vi "Start Module.vi"(6 "Show Main VI Diagram on Init (F)":bool, 8 "error in (no error)":errorcluster, 9 "DB-Engine":refnum<class "DB-Interface.lvclass">, 10 "Config Section":string, 11 "Run as Singleton? (F)":bool) -> (0 "error out":errorcluster, 1 "Wait for Event Sync?":bool, 2 "DB_CONNECTOR Broadcast Events":T1, 3 "Module ID":i32)   [LabVIEW 2022 SP3, in "hse-db.lvlib" / "DB_CONNECTOR.lvlib"]
doc: "Launches the Module Main.vi.\n____\nHAMPEL SOFTWARE ENGINEERING v1.4.0 (2023-12-19 09:52)"
uses:
  DB_CONNECTOR.lvlib
  Broadcast Events--cluster.ctl
  Did Init Argument--cluster.ctl
  Status Updated Argument--cluster.ctl
  Error Reported Argument--cluster.ctl
  Stop Argument--cluster.ctl
  Get Module Execution Status Argument--cluster.ctl
  Fast Query Reply Argument--cluster.ctl
  Configured and Connected Argument--cluster.ctl
  DB-Interface/DB-Interface.lvclass
  Module Running State--enum.ctl
  <vilib>/Delacor/Delacor QMH/Libraries/Cloneable Module Admin_class/Delacor_lib_QMH_Cloneable Module Admin.lvclass
  C:/Program Files/National Instruments/LabVIEW 2022/vi.lib/Delacor/Delacor QMH/Libraries/Module Admin_class/Delacor_lib_QMH_Module Admin.lvclass
  VI Reference Management/Main VI Type--strict_vi_ref.ctl
  <vilib>/Delacor/Delacor QMH/Libraries/Cloneable Module Admin_class/Delacor_lib_QMH_Cloneable Module Admin.lvclass/Delacor_lib_QMH_Cloneable Module Admin.ctl
  <vilib>/Delacor/Delacor QMH/Libraries/Module Admin_class/Delacor_lib_QMH_Module Admin.lvclass/Delacor_lib_QMH_Module Admin.ctl
  <vilib>/Delacor/Delacor QMH/Libraries/Cloneable Module Admin_class/Delacor_lib_QMH_Set Module ID.vi
  <vilib>/Delacor/Delacor QMH/Libraries/Module Admin_class/Delacor_lib_QMH_Set External Launch.vi
  Main.vi
  <vilib>/Utility/error.llb/Error Cluster From Error Code.vi
  <vilib>/ErrorRing/Error Ring.xnode
  Clone Registration/Clone Registration.lvlib
  VI Reference Management/VI Reference Management.lvlib
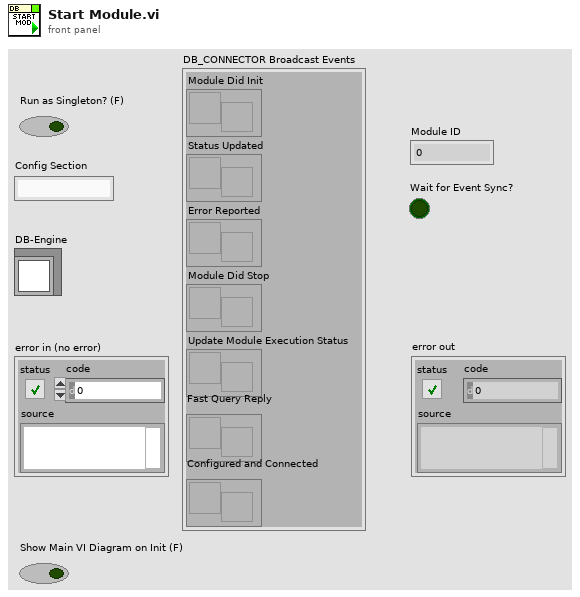
[diagram p1: front panel]
types:
  T1 = typedef "hse-db.lvlib/DB_CONNECTOR.lvlib/Broadcast Events--cluster.ctl" = cluster{"Module Did Init":refnum<user-event>, "Status Updated":refnum<user-event>, "Error Reported":refnum<user-event>, "Module Did Stop":refnum<user-event>, "Update Module Execution Status":refnum<user-event>, "Fast Query Reply":refnum<user-event>, "Configured and Connected":refnum<user-event>}
  T2 = typedef "hse-db.lvlib/DB_CONNECTOR.lvlib/Module Running State--enum.ctl" = enum16{"Not Running", "Running as Cloneable", "Running as Singleton"}
  T3 = enum32{"Bad", "Idle", "Run top level", "Running"}
  T4 = typedef "hse-db.lvlib/DB_CONNECTOR.lvlib/VI Reference Management.lvlib/Main VI Type--strict_vi_ref.ctl" = refnum<vi>
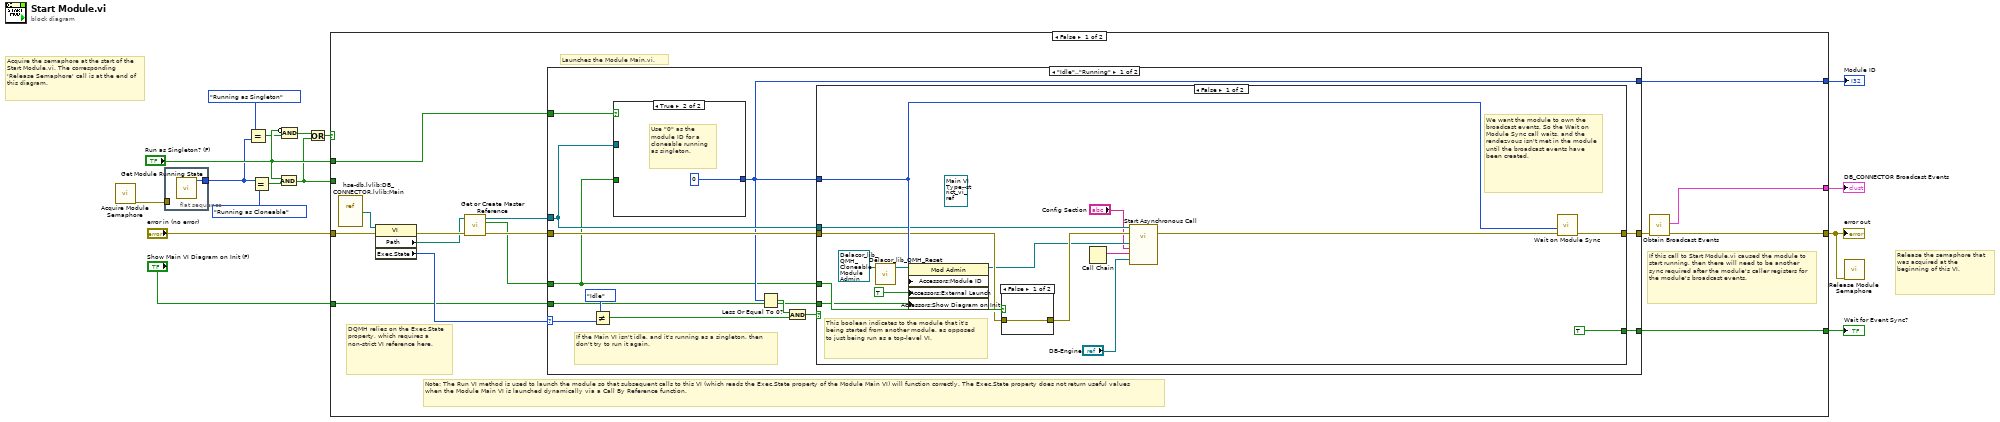
[diagram p0: block diagram]
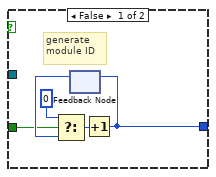
[diagram p2: hidden frame]
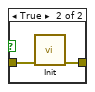
[diagram p3: hidden frame]
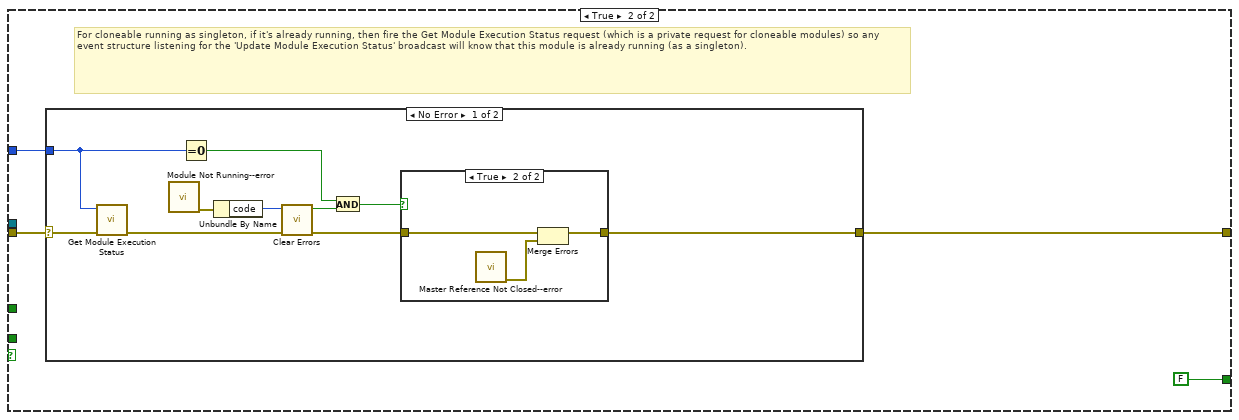
[diagram p4: hidden frame]
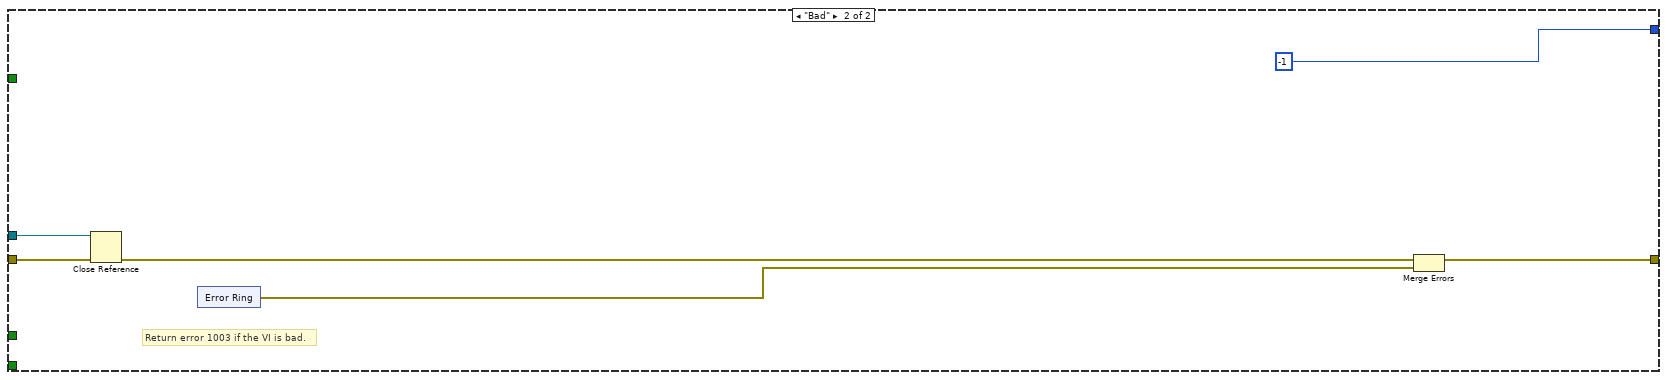
[diagram p7: hidden frame]
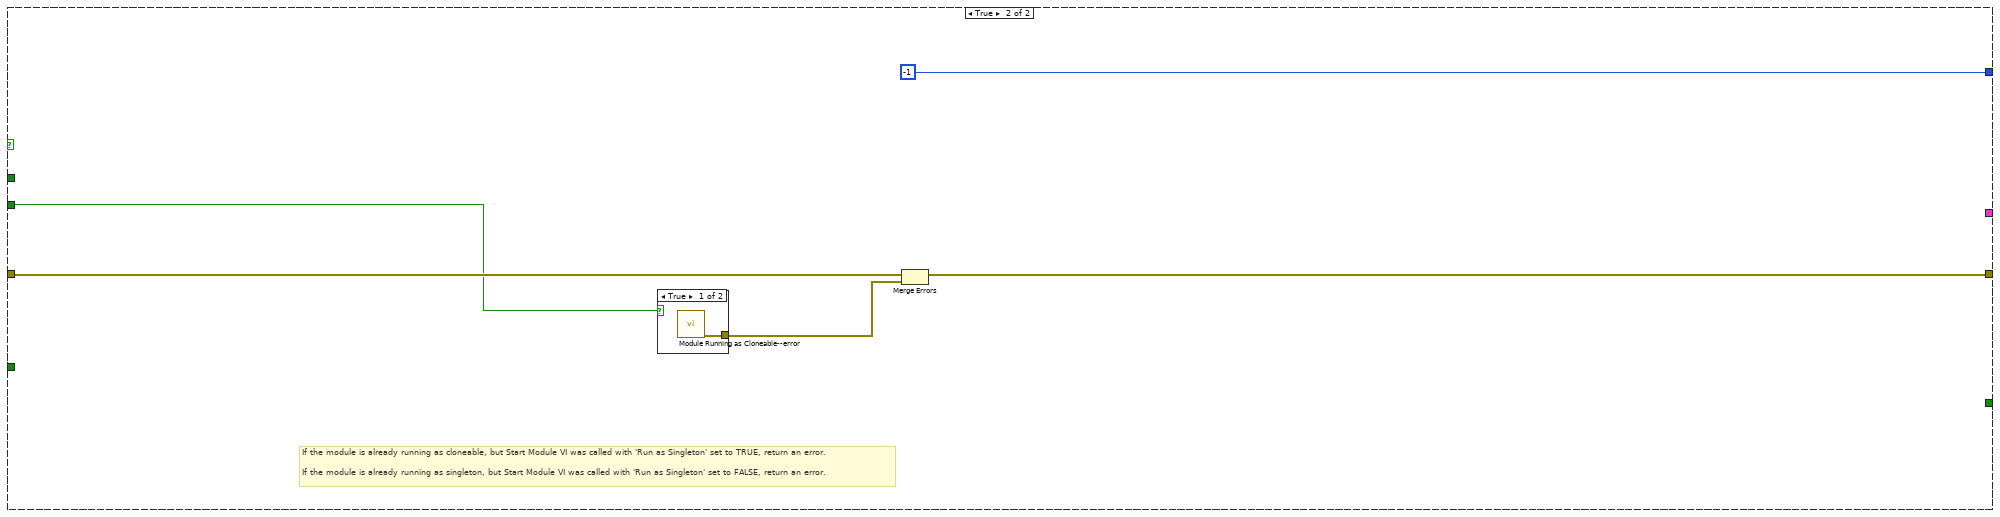
[diagram p8: hidden frame]
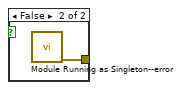
[diagram p9: hidden frame]
diagram:
  # "Release the semaphore that was acquired at the beginning of this VI."
  # "Acquire the semaphore at the start of the Start Module.vi. The corresponding 'Release Semaphore' call is at the end of this diagram."
  n1 = call "Acquire Module Semaphore.vi"() -> ("error out"=w3:errorcluster)  [unwired: 11 in]
  n2 = flat-sequence {
    tunnel: [w17] -> w6
    tunnel: w3 -> [_]
    frame #0 {
      n3 = call "Get Module Running State.vi"() -> ("Module Running State"=w17:T2)  [unwired: 11 in]
    }
  }
  n4 = Equal?(x=Module_Running_State--enum."Running as Singleton", y=w6) -> (x = y?=w7:bool)
  n5 = Equal?(x=w6, y=Module_Running_State--enum."Running as Cloneable") -> (x = y?=w11:bool)
  n6 = And(x="Run as Singleton? (F)", y=w11) -> (x .and. y?=w4:bool)
  n7 = Compound Arithmetic op=AND(invert "Run as Singleton? (F)", w7) -> (w9:bool)
  n8 = Or(x=w9, y=w4) -> (x .or. y?=w10:bool)
  n9 = case shown="False" w10 {
    tunnel: "error in (no error)" -> [w32 w104]
    tunnel: [w30 w103] -> w2
    tunnel: [w29 _] -> w15
    tunnel: [w28 _] -> w14
    tunnel: [w27 -1] -> w13
    tunnel: "Run as Singleton? (F)" -> [w24 _]
    tunnel: w4 -> [_ w100]
    tunnel: "Show Main VI Diagram on Init (F)" -> [w18 _]
    frame False {
      # "DQMH relies on the Exec.State property, which requires a non-strict VI reference here."
      # "Note: The Run VI method is used to launch the module so that subsequent calls to this VI (which reads the Exec.State property of the Module Main VI) will function correctly. The Exec.State property does not return useful values when the Module Main VI is launched dynamically via a Call By Reference function."
      # "If this call to Start Module.vi caused the module to start running, then there will need to be another sync required after the module's caller registers for the module's broadcast events."
      # "Launches the Module Main.vi."
      n10 = vi-ref "hse-db.lvlib:DB_CONNECTOR.lvlib:Main.vi"() -> (w26:refnum<vi>)
      n11 = property class="VI"(reference=w26, error in=w32) -> (error out=w23:errorcluster, "Path"=w22:path, "Exec.State"=w25:T3)  [unwired: 1 out]
      n12 = call "Get or Create Master Reference.vi"("error in (no error)"=w23, "Main VI Path"=w22) -> ("error out"=w21:errorcluster, "New Reference Created"=w19:bool, "Master Reference"=w20:T4)  [unwired: 7 in]
      n13 = case shown="\"Idle\"..\"Running\"" w25 {
        selector: w25 -> [w41 _]
        tunnel: w21 -> [w45 w95]
        tunnel: w20 -> [w43 w94]
        tunnel: [w42 w92] -> w31
        tunnel: [w44 _] -> w28
        tunnel: [w36 -1] -> w27
        tunnel: w24 -> [w35 _]
        tunnel: w19 -> [w34 _]
        tunnel: w18 -> [w33 _]
        frame "Idle".."Running" {
          # "If the Main VI isn't idle, and it's running as a singleton, then don't try to run it again."
          n14 = Not Equal?(x=T3."Idle", y=w41) -> (x != y?=w39:bool)
          n15 = case shown="True" w35 {
            tunnel: w43 -> [_ _]
            tunnel: [w47 0] -> w36
            tunnel: w34 -> [w46 _]
            frame False {
              # "generate module ID"
              n16 = feedback #1() -> (w49:i32)  [unwired: 1 in]
              n17 = Select(t=0, s=w46, f=w49) -> (s? t:f=w50:i32)
              n18 = Increment(x=w50) -> (x+1=w47:i32)
              n19 = feedback-in #1(w47) -> ()
            }
            frame True {
              # "Use \"0\" as the module ID for a cloneable running as singleton."
            }
          }
          n20 = Less Or Equal To 0?(x=w36) -> (x <= 0?=w37:bool)
          n21 = And(x=w37, y=w39) -> (x .and. y?=w38:bool)
          n22 = case shown="False" w38 {
            tunnel: w45 -> [w60 w71]
            tunnel: [TRUE FALSE] -> w44
            tunnel: w43 -> [w58 _]
            tunnel: [w66 w72] -> w42
            tunnel: w36 -> [w62 w73]
            tunnel: w34 -> [w61 _]
            tunnel: w33 -> [w52 _]
            frame False {
              (unwired) T4 refnum ("Main VI Type")
              # "We want the module to own the broadcast events. So the Wait on Module Sync call waits, and the rendezvous isn't met in the module until the broadcast events have been created."
              # "This boolean indicates to the module that it's being started from another module, as opposed to just being run as a top-level VI."
              n23 = call-dynamic "Delacor_lib_QMH_Reset.vi"("Mod Admin in"=refnum<class "Delacor_lib_QMH_Cloneable Module Admin.lvclass"> refnum) -> ("Mod Admin out"=w65:refnum<class "Delacor_lib_QMH_Cloneable Module Admin.lvclass">)  [unwired: 9 in, 1 out]
              n24 = property class="Mod Admin"(reference=w65, "Accessors:Module ID"=w62, "Accessors:External Launch"=TRUE, "Accessors:Show Diagram on Init"=w52) -> (reference out=w57:refnum<class "Delacor_lib_QMH_Cloneable Module Admin.lvclass">)  [unwired: 1 in, 1 out]
              n25 = case shown="False" w61 {
                tunnel: w60 -> [w68 w70]
                tunnel: [w68 w69] -> w59
                frame False {
                }
                frame True {
                  n26 = call "Init.vi"("error in (no error)"=w70) -> ("error out"=w69:errorcluster)  [unwired: 7 in, 3 out]
                }
              }
              n27 = Call Chain() -> (call chain=w54:string[])
              n28 = call-by-ref "Start Asynchronous Call"(reference=w58, error in=w59, "DB-Interface"="DB-Engine", "Call Chain"=w54, "Config Section"="Config Section", "Module Admin"=w57) -> (error out=w56:errorcluster)  [unwired: 8 in, 1 out]
              n29 = call "Wait on Module Sync.vi"("error in (no error)"=w56, "Module ID"=w62) -> ("error out"=w66:errorcluster)  [unwired: 9 in]
            }
            frame True {
              # "For cloneable running as singleton, if it's already running, then fire the Get Module Execution Status request (which is a private request for cloneable modules) so any event structure listening for the 'Update Module Execution Status' broadcast will know that this module is already running (as a singleton)."
              n30 = case shown="No Error" w71 {
                selector: w71 -> [w84 w89]
                tunnel: w73 -> [w83 _]
                tunnel: [w75 w89] -> w72
                frame No Error {
                  n31 = call "Get Module Execution Status.vi"("error in (no error)"=w84, "Module ID"=w83) -> ("error out"=w82:errorcluster)  [unwired: 9 in]
                  n32 = call "Module Not Running--error.vi"() -> ("error out"=w81:errorcluster)  [unwired: 11 in]
                  n33 = Equal To 0?(x=w83) -> (x = 0?=w78:bool)
                  n34 = Unbundle By Name(w81) -> ("code"=w80:i32)
                  n35 = call <vilib>:"Clear Errors.vi"("error in (no error)"=w82, "specific error code to clear (0: all)"=w80) -> ("error out"=w76:errorcluster, "specific error cleared?"=w79:bool)  [unwired: 4 in]
                  n36 = And(x=w78, y=w79) -> (x .and. y?=w77:bool)
                  n37 = case shown="True" w77 {
                    tunnel: w76 -> [w85 w87]
                    tunnel: [w85 w86] -> w75
                    frame False {
                    }
                    frame True {
                      n38 = call "Master Reference Not Closed--error.vi"() -> ("error out"=w88:errorcluster)  [unwired: 11 in]
                      n39 = Merge Errors(w87, w88) -> (w86:errorcluster)
                    }
                  }
                }
                frame Error {
                }
              }
            }
          }
        }
        frame "Bad" {
          # "Return error 1003 if the VI is bad."
          n40 = Close Reference(reference=w94, error in (no error)=w95) -> (error out=w93:errorcluster)
          n41 = xnode "Error Ring"() -> ("error out"=w91:errorcluster)
          n42 = Merge Errors(w93, w91) -> (w92:errorcluster)
        }
      }
      n43 = call "Obtain Broadcast Events.vi"("error in (no error)"=w31) -> ("error out"=w30:errorcluster, "DB_CONNECTOR Broadcast Events"=w29:T1)  [unwired: 9 in]
    }
    frame True {
      # "If the module is already running as cloneable, but Start Module VI was called with 'Run as Singleton' set to TRUE, return an error.\n\nIf the module is already running as singleton, but Start Module VI was called with 'Run as Singleton' set to FALSE, return an error."
      n44 = case shown="True" w100 {
        tunnel: [w105 w106] -> w101
        frame True {
          n45 = call "Module Running as Cloneable--error.vi"() -> ("error out"=w105:errorcluster)  [unwired: 11 in]
        }
        frame False {
          n46 = call "Module Running as Singleton--error.vi"() -> ("error out"=w106:errorcluster)  [unwired: 11 in]
        }
      }
      n47 = Merge Errors(w104, w101) -> (w103:errorcluster)
    }
  }
  "error out" <- w2
  "DB_CONNECTOR Broadcast Events" <- w15
  "Wait for Event Sync?" <- w14
  "Module ID" <- w13
  n48 = call "Release Module Semaphore.vi"("error in (no error)"=w2) -> ()  [unwired: 10 in, 1 out]
